vi "Render Ship In Sidebar.vi"(7 "Renderer":refnum<class "Renderer.lvclass">, 8 "error in (no error)":errorcluster, 11 "Ship in":refnum<class "Ship.lvclass">) -> (0 "error out":errorcluster)   [LabVIEW 2021, in "Ship.lvclass"]
uses:
  Ship.lvclass
  C:/dev/LabVIEW/LabMelee/Source/Application Specific/Element/Element.lvclass
  Renderer/Renderer.lvclass
  Element/Element.lvclass/Element.ctl
  Ship.lvclass/Ship.ctl
  Texture/Texture.lvclass/Texture.ctl
  Re-use Libraries/Vector 2D/Vector 2D.lvclass/Vector 2D.ctl
  Renderer/Renderer.lvclass/Renderer.ctl
  Re-use Libraries/Vector 2D/Vector 2D.lvclass
  Resource Manager/Resource Manager.lvclass
  Element/Element.lvclass
  Texture/Texture.lvclass
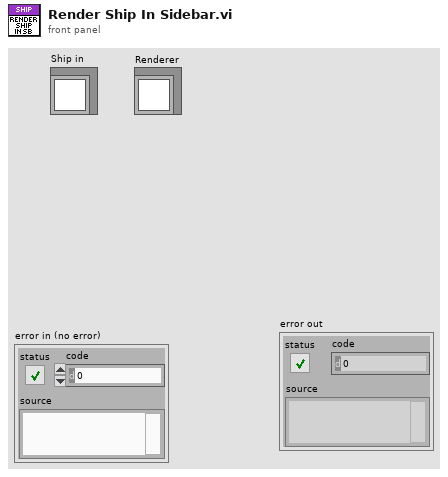
[diagram p1: front panel]
types:
  T1 = typedef "Element.lvclass/Player Type.ctl" = enum16{"Neutral", "Player 1", "Player 2"}
  T2 = typedef "Constants.ctl" = cluster{"Colours":cluster{"OK":u32, "Warning":u32, "Error":u32, "Red":u32, "Green":u32, "Blue":u32, "Yellow":u32}, "System":cluster{"Target Frames Second":dbl, "World Size":T3, "Window Size":T3, "Battle Area Size":T3, "Sidebar Width":sgl, "SC2 Frame Rate [Seconds/Frame]":sgl, "Sidebar Player 2 Y Offset":sgl, "Windows Size V2":refnum<class "Vector 2D.lvclass">, "World Size V2":refnum<class "Vector 2D.lvclass">, "Battle Area Size V2":refnum<class "Vector 2D.lvclass">}, "Game":cluster{"Maximum Asteroids":i32, "Max Energy":i32, "Max Crew":i32, "Maximum Stars":i32}}
  T3 = typedef "SDL2 Utility.lvlib/Point (I32).ctl" = cluster{"x":i32, "y":i32}
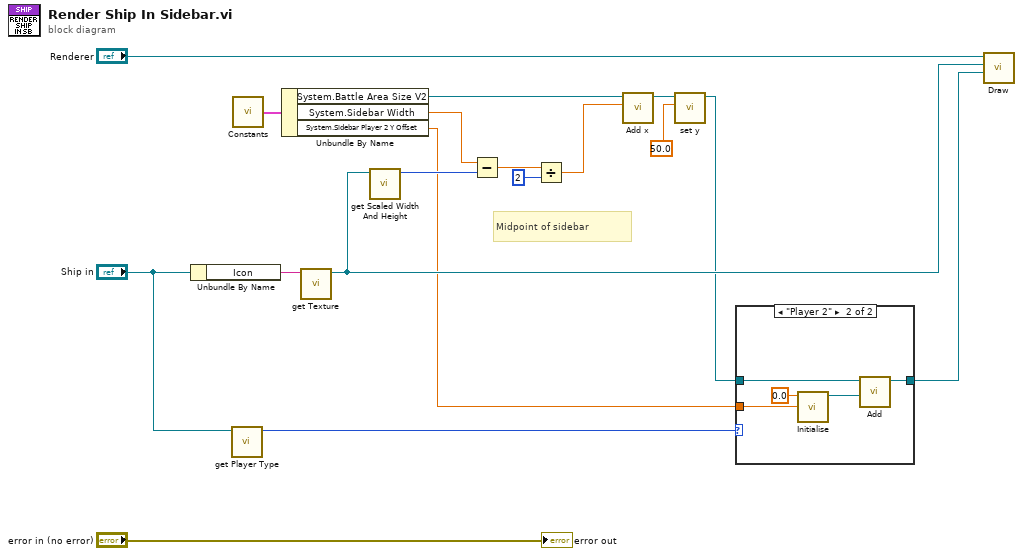
[diagram p0: block diagram]
diagram:
  # "Midpoint of sidebar"
  n1 = Unbundle By Name("Ship in") -> ("Icon"=w17:string)
  n2 = call "get Player Type.vi"("Element in"="Ship in") -> ("Player Type"=w15:T1)  [unwired: 10 in]
  n3 = call "Constants.vi"() -> ("Constants"=w18:T2)
  n4 = Unbundle By Name(w18) -> ("System.Battle Area Size V2"=w6:refnum<class "Vector 2D.lvclass">, "System.Sidebar Width"=w11:sgl, "System.Sidebar Player 2 Y Offset"=w1:sgl)
  n5 = call "get Texture.vi"("Texture Name"=w17) -> ("Texture"=w12:refnum<class "Texture.lvclass">)  [unwired: 10 in]
  n6 = call "get Scaled Width And Height.vi"("Texture in"=w12) -> ("Width"=w10:i32)  [unwired: 9 in, 1 out]
  n7 = Subtract(x=w11, y=w10) -> (x-y=w9:sgl)
  n8 = Divide(x=w9, y=2) -> (x/y=w5:sgl)
  n9 = call "Add x.vi"("x"=w5, "Vector 2D in"=w6) -> ("Vector 2D out"=w4:refnum<class "Vector 2D.lvclass">)  [unwired: 9 in]
  n10 = call "set y.vi"("y"=sgl 50.0 ("y 2"), "Vector 2D in"=w4) -> ("Vector 2D out"=w3:refnum<class "Vector 2D.lvclass">)  [unwired: 9 in]
  n11 = case shown="\"Player 2\"" w15 {
    tunnel: [w19 w23] -> w7
    tunnel: w3 -> [w19 w24]
    tunnel: w1 -> [_ w20]
    frame "Player 1", Default {
    }
    frame "Player 2" {
      n12 = call "Initialise.vi"("y"=w20, "x"=sgl 0.0) -> ("Vector 2D out"=w21:refnum<class "Vector 2D.lvclass">)  [unwired: 9 in]
      n13 = call "Add.vi"("B"=w21, "A"=w24) -> ("A+B"=w23:refnum<class "Vector 2D.lvclass">)  [unwired: 9 in]
    }
  }
  n14 = call "Draw.vi"("Destination"=w7, "Texture"=w12, "Renderer"="Renderer") -> ()  [unwired: 8 in, 1 out]
  "error out" <- "error in (no error)"
